vi "LWXPS_ObjectsListGet.vi"(0 "XPS Reference IN":refnum<k24>, 11 "LabVIEW error IN":errorcluster) -> (4 "XPS Reference OUT":refnum<k24>, 6 "Returned error code":i32, 8 "Objects List":string, 10 "XPS Error String":string, 15 "LabVIEW error OUT":errorcluster)   [LabVIEW 2014]
uses:
  D:/XPSQ8_LabView_Library/Development/Source/Dll/Newport.XPS.CommandInterface.dll
  Dll/Newport.XPS.CommandInterface.dll
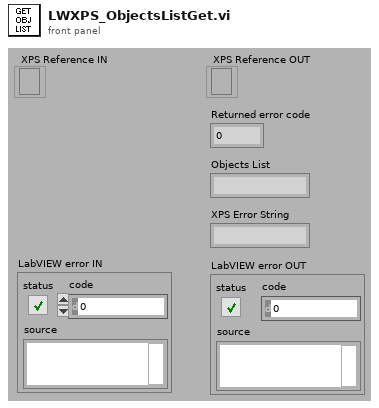
[diagram p1: front panel]
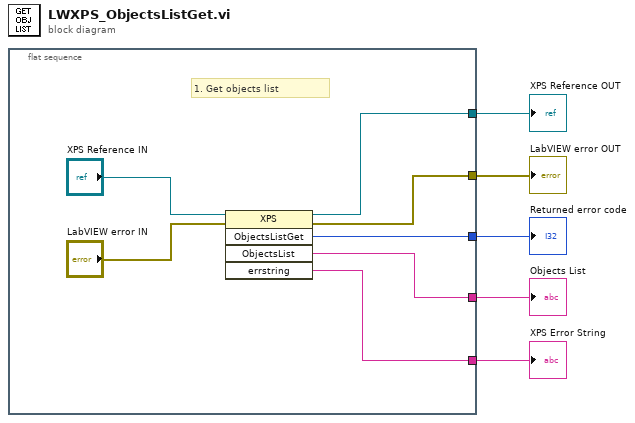
[diagram p0: block diagram]
diagram:
  n1 = flat-sequence {
    tunnel: [w11] -> w1
    tunnel: [w10] -> w5
    tunnel: [w9] -> w4
    tunnel: [w8] -> w3
    tunnel: [w7] -> w2
    frame #0 {
      # "1. Get objects list"
      n2 = invoke class="XPS" method="ObjectsListGet"(reference="XPS Reference IN", error in="LabVIEW error IN") -> (reference out=w9:refnum<k24>, error out=w8:errorcluster, "ObjectsListGet"=w7:i32, "ObjectsList"=w11:string, "errstring"=w10:string)  [unwired: 3 in]
    }
  }
  "XPS Error String" <- w5
  "XPS Reference OUT" <- w4
  "LabVIEW error OUT" <- w3
  "Returned error code" <- w2
  "Objects List" <- w1
